vi "Phase shift check.vi"(7 "Half period":i32=5, 11 "Wave form":i16[](array[numeric])) -> (2 "theta":dbl[](array[numeric]), 3 "r":dbl[](array[numeric]))   [LabVIEW 2014]
uses:
  <vilib>/Analysis/NI_AALPro.lvlib
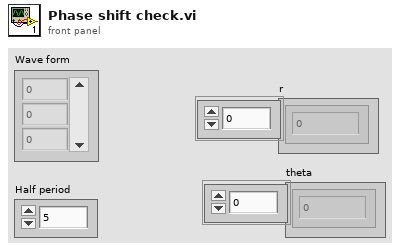
[diagram p1: front panel]
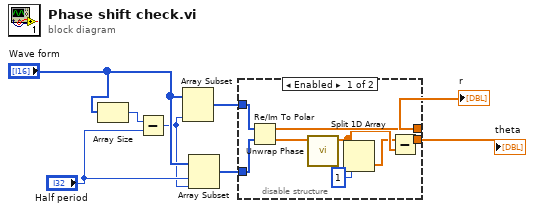
[diagram p0: block diagram]
diagram:
  n1 = Array Size(array="Wave form") -> (size(s)=w8:i32)
  n2 = Subtract(x=w8, y="Half period") -> (x-y=w5:i32)
  n3 = Array Subset(array="Wave form", length=w5) -> (w4:i16[])  [unwired: 1 in]
  n4 = Array Subset(array="Wave form", index="Half period", length=w5) -> (w3:i16[])
  n5 = disable-structure shown="Enabled" {
    disable-tunnel: w4 -> [w16 w18]
    disable-tunnel: w3 -> [w15 w17]
    disable-tunnel: [w14 w18] -> w2
    disable-tunnel: [w11 w17] -> w1
    frame Enabled {
      n6 = Re/Im To Polar(2:w15, 3:w16) -> (0:w13:dbl[], 1:w14:dbl[])
      n7 = call <vilib>:"Unwrap Phase.vi"("Phase"=w13) -> ("Unwrapped Phase"=w10:dbl[])  [unwired: 9 in, 1 out]
      n8 = Split 1D Array(array=w10, index=1) -> (second subarray=w9:dbl[])  [unwired: 1 out]
      n9 = Subtract(x=w9, y=w10) -> (x-y=w11:dbl[])
    }
    frame Disabled {
    }
  }
  "r" <- w2
  "theta" <- w1
